vi "Read Tree Menu Plugin Entries.vi"(4 "Error In":errorcluster, 6 "Menu Context":T1, 7 "Config Data in":refnum<class "Config Data.lvclass">) -> (0 "Error Out":errorcluster, 2 "Tree Menu Plugin Entries":T2[](array[typedef]), 3 "Config Data out":refnum<class "Config Data.lvclass">)   [LabVIEW 2020, in "Config Data.lvlib" / "Config Data.lvclass"]
uses:
  Config Data.lvclass
  typedefs/Tree Menu Entry.ctl
  typedefs/Menu Context Selections.ctl
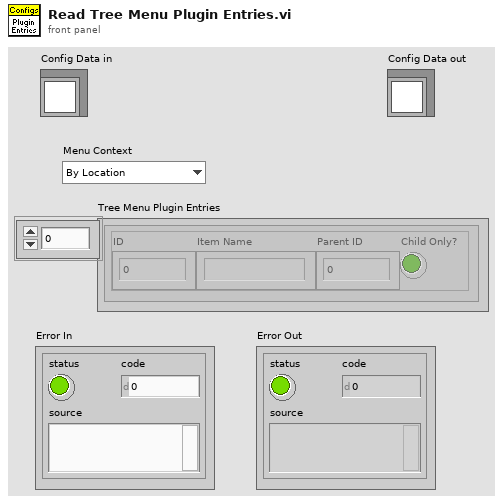
[diagram p1: front panel]
types:
  T1 = typedef "Config Data.lvlib/Config Data.lvclass/Menu Context Selections.ctl" = enum16{"By Location", "By Function"}
  T2 = typedef "Config Data.lvlib/Config Data.lvclass/Tree Menu Entry.ctl" = cluster{"ID":i32, "Item Name":string, "Parent ID":i32, "Child Only?":bool}
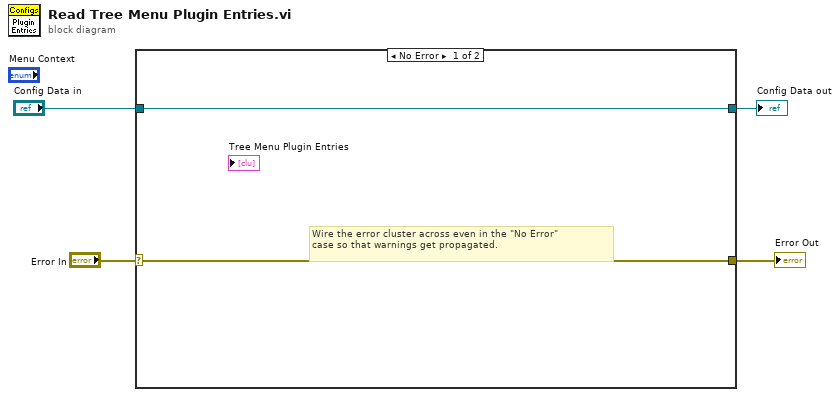
[diagram p0: block diagram]
diagram:
  n1 = case shown="No Error" "Error In" {
    selector: "Error In" -> [w5 w8]
    tunnel: [w5 w8] -> w1
    tunnel: [w6 w7] -> w3
    tunnel: "Config Data in" -> [w6 w7]
    frame No Error {
      # "Wire the error cluster across even in the \"No Error\"\ncase so that warnings get propagated."
    }
    frame Error {
    }
  }
  "Config Data out" <- w3
  "Error Out" <- w1
